vi "test_DependencyList_InsertNewItem.vi"() -> (3 "Pass?":bool)   [LabVIEW 2020, in "Tests.DependencyInspection.lvlib"]
uses:
  Tests.DependencyInspection.lvlib
  CDependencyList/CDependencyList.lvclass
  ItemInfo.ctl
  obj/Addons/LabVIEWObjectInterfaces.lvlibp/LabVIEWObjectInterfaces/ILabVIEWItem/ILabVIEWItem.lvclass
  obj/Addons/LabVIEWObjectFactory.lvlibp
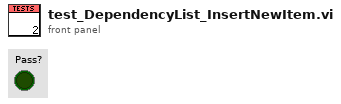
[diagram p1: front panel]
types:
  T1 = typedef "Tests.DependencyInspection.lvlib/ItemInfo.ctl" = cluster{"path":path, "delimited name":string}
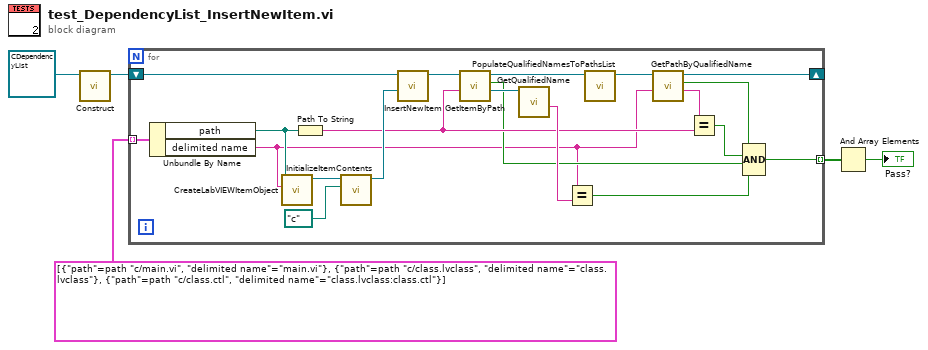
[diagram p0: block diagram]
diagram:
  n1 = call-dynamic "Construct.vi"("CDependencyList in"=refnum<class "CDependencyList.lvclass"> refnum) -> ("CDependencyList out"=w1:refnum<class "CDependencyList.lvclass">)  [unwired: 9 in, 1 out]
  n2 = for {
    tunnel: [w14] -> w5 mode=indexing
    tunnel: T1[] [{"path"=path "c:/main.vi", "delimited name"="main.vi"}, {"path"=path "c:/class.lvclass", "delimited name"="class.lvclass"}, {"path"=path "c:/class.ctl", "delimited name"="class.lvclass:class.ctl"}] -> [w10] mode=indexing
    shift-right: [w7] -> _
    shift-left: w1 -> [w6]
    n3 = Unbundle By Name(w10) -> ("path"=w9:path, "delimited name"=w8:string)
    n4 = call "CreateLabVIEWItemObject.vi"("delimited name"=w8, "SubVI path"=w9) -> ("ILabVIEWItem"=w25:refnum<class "ILabVIEWItem.lvclass">)  [unwired: 8 in, 1 out]
    n5 = Path To String(path=w9) -> (string=w16:string)
    n6 = call-dynamic "InitializeItemContents.vi"("Root path"=path "c:/", "ILabVIEWItem in"=w25) -> ("ILabVIEWItem out"=w23:refnum<class "ILabVIEWItem.lvclass">)  [unwired: 8 in, 1 out]
    n7 = call-dynamic "InsertNewItem.vi"("ILabVIEWItem in"=w23, "CDependencyList in"=w6) -> ("CDependencyList out"=w22:refnum<class "CDependencyList.lvclass">)  [unwired: 7 in, 2 out]
    n8 = call-dynamic "GetItemByPath.vi"("Path"=w16, "CDependencyList in"=w22) -> ("ILabVIEWItem"=w19:refnum<class "ILabVIEWItem.lvclass">, "key found?"=w11:bool, "CDependencyList out"=w21:refnum<class "CDependencyList.lvclass">)  [unwired: 6 in, 1 out]
    n9 = call-dynamic "GetQualifiedName.vi"("ILabVIEWItem in"=w19) -> ("Qualified name"=w18:string)  [unwired: 8 in, 2 out]
    n10 = Equal?(x=w8, y=w18) -> (x = y?=w12:bool)
    n11 = call-dynamic "PopulateQualifiedNamesToPathsList.vi"("CDependencyList in"=w21) -> ("CDependencyList out"=w20:refnum<class "CDependencyList.lvclass">)  [unwired: 9 in, 1 out]
    n12 = call-dynamic "GetPathByQualifiedName.vi"("Qualified name"=w8, "CDependencyList in"=w20) -> ("Path"=w17:string, "key found?"=w13:bool, "CDependencyList out"=w7:refnum<class "CDependencyList.lvclass">)  [unwired: 6 in, 1 out]
    n13 = Equal?(x=w17, y=w16) -> (x = y?=w15:bool)
    n14 = Compound Arithmetic op=AND(w13, w15, w11, w12) -> (w14:bool)
  }
  n15 = And Array Elements(Boolean array=w5) -> (logical AND=→"Pass?":bool)
